vi "PTSequencer.DIM update.vi"(0 "i ref in":refnum<vi>, 1 "data":i8[](array[numeric]), 2 "serviceName":string, 5 "error in (no error)":errorcluster, 6 "Time Stamp":dbl, 7 "no link":bool, 8 "quality":i32) -> (14 "i ref out":refnum<vi>, 19 "error out":errorcluster)   [LabVIEW 2014, in "PTSequencer.lvlib"]
uses:
  PTSequencer.lvlib
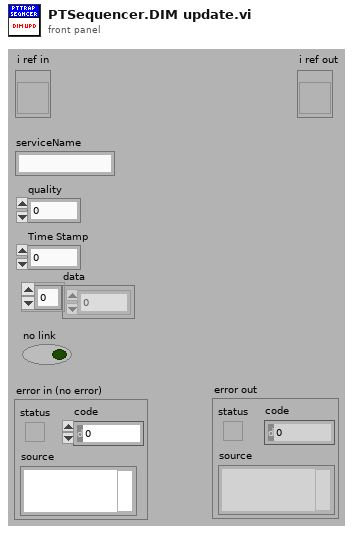
[diagram p1: front panel]
types:
  T1 = typedef "PTSequencer.lvlib/PTSequencer.i attribute.ctl" = cluster{"subsequence":bool, "mode":T2, "i step":i32, "nofLoops":i32, "i loop":i32, "Running":bool, "Paused":bool, "step done":bool, "loop done":bool, "seq done":bool, "DIM IDs":cluster{"step done":i32, "loop done":i32, "seq done":i32, "i step":i32, "i loop":i32}, "use stop conditions":bool, "stop conditions":T3[], "Step List":T5[], "DIM subsriptions":string[], "stop cond indexes":i32[], "step cond indexes":cluster{"step condition IDs":cluster{"step ID":i32, "condition ID":i32}[]}[], "Delay Start Time":timestamp, "status":string, "stopping":bool}
  T2 = typedef "PTSequencer.lvlib/PTSequencer.mode.ctl" = enum16{"single", "loop", "for loop"}
  T3 = typedef "PTSequencer.lvlib/PTSequencer.DIM service condition.ctl" = cluster{"DIM service":string, "descr":string, "nomValue":T4, "actValue":T4, "matched":bool, "DIM Status":cluster{"no link":bool, "quality":i32, "Time Stamp":timestamp}}
  T4 = typedef "CoreDefs.rawDataType.ctl" = i8[]
  T5 = typedef "PTSequencer.lvlib/PTSequencer.step.ctl" = cluster{"description":string, "object parameters":cluster{"object":string, "selector":string, "descriptor":string, "data":T4, "subsequence":bool, "call mode":enum16{"Simple DIM", "Synchronous"}, "data in":T4}, "result action":cluster{"check":bool, "passed":enum16{"Next", "Previous", "Repeat", "Jump"}, "failed":enum16{"Next", "Previous", "Repeat", "Jump"}, "jumpID_passed":i32, "jumpID_failed":i32}, "conditions":T3[], "fulfilled ":bool, "use delay":bool, "delay time (s)":dbl, "ID":i32}
  T6 = cluster{"step condition IDs":cluster{"step ID":i32, "condition ID":i32}[]}[]
  T7 = cluster{"step condition IDs":cluster{"step ID":i32, "condition ID":i32}[]}
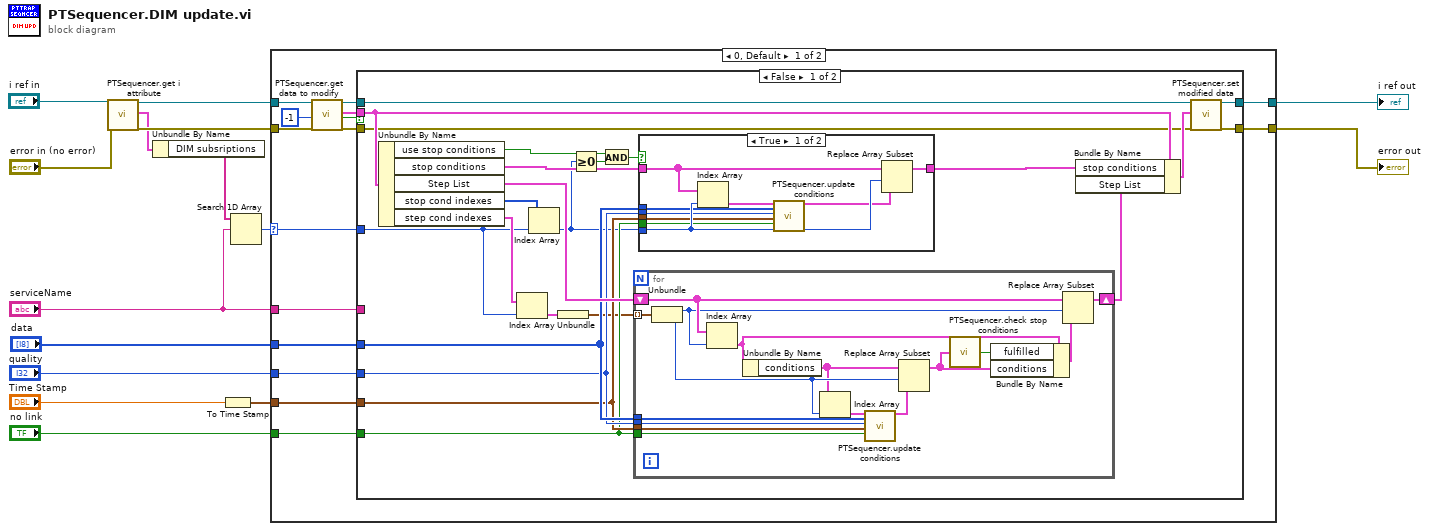
[diagram p0: block diagram]
diagram:
  n1 = call "PTSequencer.get i attribute.vi"("i ref in"="i ref in", "error in (no error)"="error in (no error)") -> ("i ref out"=w14:refnum<vi>, "i attribute"=w12:T1, "error out"=w13:errorcluster)  [unwired: 15 in]
  n2 = Unbundle By Name(w12) -> ("DIM subsriptions"=w2:string[])
  n3 = To Time Stamp(1:"Time Stamp") -> (0:w15:timestamp)
  n4 = Search 1D Array(1D array=w2, element="serviceName") -> (index of element=w3:i32)  [unwired: 1 in]
  n5 = case shown="0, Default" w3 {
    selector: w3 -> [w16 _]
    tunnel: [w26 w82] -> w5
    tunnel: [w25 w83] -> w11
    tunnel: "data" -> [w24 _]
    tunnel: "quality" -> [w23 _]
    tunnel: w15 -> [w22 _]
    tunnel: "no link" -> [w21 _]
    tunnel: w14 -> [w20 w83]
    tunnel: w13 -> [w18 w82]
    tunnel: "serviceName" -> [w17 _]
    frame 0, Default {
      n6 = call "PTSequencer.get data to modify.vi"("i ref in"=w20, "ms timeout (10000)"=-1, "error in (no error)"=w18) -> ("i ref out"=w28:refnum<vi>, "i attribute"=w29:T1, "timed out"=w30:bool, "error out"=w27:errorcluster)  [unwired: 13 in]
      n7 = case shown="False" w30 {
        tunnel: w29 -> [w49 _]
        tunnel: w28 -> [w51 w80]
        tunnel: [w53 w81] -> w26
        tunnel: w27 -> [w48 w81]
        tunnel: [w52 w80] -> w25
        tunnel: w24 -> [w39 _]
        tunnel: w23 -> [w38 _]
        tunnel: w22 -> [w37 _]
        tunnel: w21 -> [w36 _]
        tunnel: w17 -> [_ _]
        tunnel: w16 -> [w45 _]
        frame False {
          n8 = Unbundle By Name(w49) -> ("use stop conditions"=w33:bool, "stop conditions"=w44:T3[], "Step List"=w41:T5[], "stop cond indexes"=w47:i32[], "step cond indexes"=w46:T6)
          n9 = Index Array(array=w46, index=w45) -> (element=w42:T7)
          n10 = Index Array(array=w47, index=w45) -> (element=w35:i32)
          n11 = Unbundle(w42) -> ("step condition IDs"=w31:cluster{"step ID":i32, "condition ID":i32}[])
          n12 = Greater Or Equal To 0?(x=w35) -> (x >= 0?=w34:bool)
          n13 = And(x=w33, y=w34) -> (x .and. y?=w32:bool)
          n14 = for {
            tunnel: w31 -> [w69] mode=indexing
            tunnel: w39 -> [w60]
            tunnel: w38 -> [w59]
            tunnel: w37 -> [w58]
            tunnel: w36 -> [w57]
            shift-right: [w63] -> w40
            shift-left: w41 -> [w67]
            n15 = Unbundle(w69) -> ("step ID"=w66:i32, "condition ID"=w68:i32)
            n16 = Index Array(array=w67, index=w66) -> (element=w65:T5)
            n17 = Unbundle By Name(w65) -> ("conditions"=w56:T3[])
            n18 = Index Array(array=w56, index=w68) -> (element=w62:T3)
            n19 = call "PTSequencer.update conditions.vi"("condition in"=w62, "data"=w60, "quality"=w59, "Time Stamp"=w58, "no link"=w57) -> ("condition out"=w61:T3)  [unwired: 14 in]
            n20 = Replace Array Subset(array=w56, new element=w61, index=w68) -> (w55:T3[])
            n21 = call "PTSequencer.check stop conditions.vi"("conditions"=w55) -> ("fulfilled"=w54:bool)
            n22 = Bundle By Name(cluster=w65, "fulfilled"=w54, "conditions"=w55) -> (w64:T5)
            n23 = Replace Array Subset(array=w67, new element=w64, index=w66) -> (w63:T5[])
          }
          n24 = case shown="True" w32 {
            tunnel: w44 -> [w78 w79]
            tunnel: w35 -> [w77 _]
            tunnel: [w76 w79] -> w43
            tunnel: w39 -> [w73 _]
            tunnel: w38 -> [w72 _]
            tunnel: w37 -> [w71 _]
            tunnel: w36 -> [w70 _]
            frame True {
              n25 = Index Array(array=w78, index=w77) -> (element=w75:T3)
              n26 = call "PTSequencer.update conditions.vi"("condition in"=w75, "data"=w73, "quality"=w72, "Time Stamp"=w71, "no link"=w70) -> ("condition out"=w74:T3)  [unwired: 14 in]
              n27 = Replace Array Subset(array=w78, new element=w74, index=w77) -> (w76:T3[])
            }
            frame False {
            }
          }
          n28 = Bundle By Name(cluster=w49, "stop conditions"=w43, "Step List"=w40) -> (w50:T1)
          n29 = call "PTSequencer.set modified data.vi"("i ref in"=w51, "CLASS.i attribute"=w50, "error in (no error)"=w48) -> ("i ref out"=w52:refnum<vi>, "error out"=w53:errorcluster)  [unwired: 15 in]
        }
        frame True {
        }
      }
    }
    frame -1 {
    }
  }
  "i ref out" <- w11
  "error out" <- w5
